vi "Waveform_shift.vi"(9 "Delay (ns)":dbl, 10 "Attenuation":dbl, 11 "Waveform_in":waveform(dbl)[](array[waveform])) -> (3 "Wavefrom_out":waveform(dbl)[](array[waveform]))   [LabVIEW 2019]
uses:
  <vilib>/Analysis/3filter.llb/Savitzky-Golay Filter (DBL).vi
  <vilib>/Analysis/NI_AALBase.lvlib
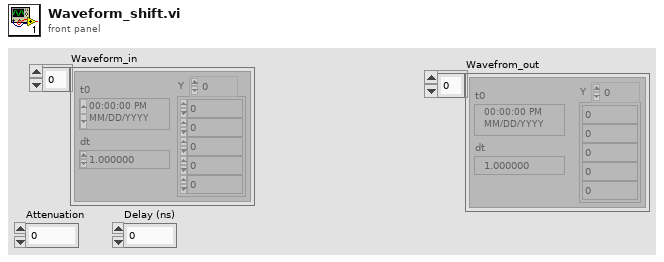
[diagram p1: front panel]
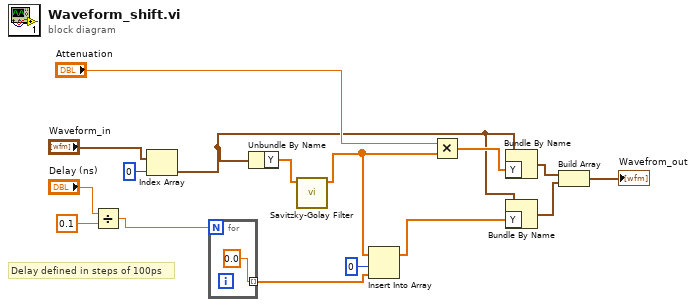
[diagram p0: block diagram]
diagram:
  # "Delay defined in steps of 100ps"
  n1 = Divide(x="Delay (ns)", y=0.1) -> (x/y=w8:dbl)
  n2 = Index Array(array="Waveform_in", index=0) -> (element=w5:waveform(dbl))
  n3 = for {
    N: w8 -> [_]
    tunnel: [0.0 ("new element/subarray")] -> w7 mode=indexing
  }
  n4 = Unbundle By Name(w5) -> ("Y"=w2:dbl[])
  n5 = call-poly <vilib>:"Savitzky-Golay Filter.vi"("X"=w2) -> ("Filtered X"=w1:dbl[])  [unwired: 9 in, 1 out]
  n6 = Insert Into Array(array=w1, index=0, new element=w7) -> (w4:dbl[])
  n7 = Multiply(x="Attenuation", y=w1) -> (x*y=w15:dbl[])
  n8 = Bundle By Name(cluster=w5, "Y"=w15) -> (w6:waveform(dbl))
  n9 = Bundle By Name(cluster=w5, "Y"=w4) -> (w3:waveform(dbl))
  n10 = Build Array(w6, w3) -> (→"Wavefrom_out":waveform(dbl)[])
